vi "Digital Meas Analyze PWM Measurements.vi"(8 "error in (no error)":errorcluster, 11 "Semiperiod Measurements (s)":dbl[](array[numeric])) -> (0 "error out":errorcluster, 3 "Digital PWM Measurements":T1 {"Duty Cycle (%)" min=0.0 max=100.0})   [LabVIEW 2024, in "NIScopeDigitalMeasurement.lvlib"]
uses:
  NIScopeDigitalMeasurement.lvlib
  Program Files (x86)/National Instruments/LabVIEW 2019/ProjectTemplates/Source/PCB Assembly Test Toolkit/Library/Digital PWM Measurement/Typedefs/Digital PWM Measurements.ctl
  <vilib>/Analysis/baseanly.llb/Mean (DBL).vi
  Program Files (x86)/National Instruments/LabVIEW 2019/ProjectTemplates/Source/PCB Assembly Test Toolkit/Library/Digital PWM Measurement/Digital PWM Measurement.lvlib
  <vilib>/Analysis/NI_AALBase.lvlib
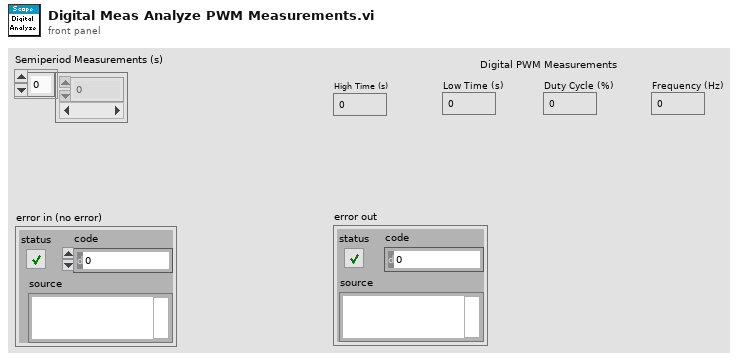
[diagram p1: front panel]
types:
  T1 = cluster{"High Time (s)":dbl, "Low Time (s)":dbl, "Duty Cycle (%)":dbl, "Frequency (Hz)":dbl}
  T2 = typedef "Digital PWM Measurement.lvlib/Digital PWM Measurements.ctl" = cluster{"High Time (s)":dbl, "Low Time (s)":dbl, "Duty Cycle (%)":dbl, "Frequency (Hz)":dbl}
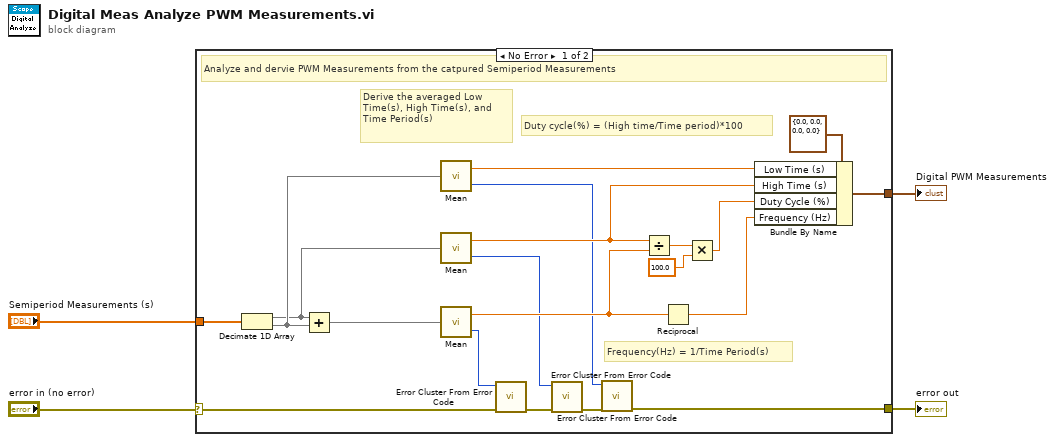
[diagram p0: block diagram]
diagram:
  n1 = case shown="No Error" "error in (no error)" {
    selector: "error in (no error)" -> [w23 w25]
    tunnel: [w22 _] -> w3
    tunnel: "Semiperiod Measurements (s)" -> [w13 _]
    tunnel: [w8 w25] -> w1
    frame No Error {
      # "Frequency(Hz) = 1/Time Period(s)"
      # "Duty cycle(%) = (High time/Time period)*100"
      # "Derive the averaged Low Time(s), High Time(s), and Time Period(s)"
      # "Analyze and dervie PWM Measurements from the catpured Semiperiod Measurements"
      n2 = Decimate 1D Array(w13) -> (w15:dbl[], w17:dbl[])
      n3 = Add(x=w15, y=w17) -> (x+y=w14:dbl[])
      n4 = call-poly <vilib>:"Mean.vi"("X"=w17) -> ("mean"=w19:dbl, "error"=w9:i32)
      n5 = call-poly <vilib>:"Mean.vi"("X"=w15) -> ("mean"=w20:dbl, "error"=w10:i32)
      n6 = call-poly <vilib>:"Mean.vi"("X"=w14) -> ("mean"=w16:dbl, "error"=w24:i32)
      n7 = call <vilib>:"Error Cluster From Error Code.vi"("error in (no error)"=w23, "error code (0)"=w24) -> ("error out"=w12:errorcluster)  [unwired: 7 in]
      n8 = call <vilib>:"Error Cluster From Error Code.vi"("error in (no error)"=w12, "error code (0)"=w10) -> ("error out"=w11:errorcluster)  [unwired: 7 in]
      n9 = call <vilib>:"Error Cluster From Error Code.vi"("error in (no error)"=w11, "error code (0)"=w9) -> ("error out"=w8:errorcluster)  [unwired: 7 in]
      n10 = Divide(x=w20, y=w16) -> (x/y=w7:dbl)
      n11 = Reciprocal(x=w16) -> (1/x=w21:dbl)
      n12 = Multiply(x=w7, y=100.0) -> (x*y=w5:dbl)
      n13 = Bundle By Name(cluster=T2 {"High Time (s)"=0.0, "Low Time (s)"=0.0, "Duty Cycle (%)"=0.0, "Frequency (Hz)"=0.0} ("Digital PWM Measurements"), "Low Time (s)"=w19, "High Time (s)"=w20, "Duty Cycle (%)"=w5, "Frequency (Hz)"=w21) -> (w22:T2)
    }
    frame Error {
      # "Error case - Post analysis for the digittal PWM Measurement is skipped"
    }
  }
  "error out" <- w1
  "Digital PWM Measurements" <- w3
